vi "Display Soft Trigger Status.vi"(11 "Soft Trig enum":T1(ring)) -> (3 "String":string)   [LabVIEW 2016, in "CML UI.lvlib"]
uses:
  CML UI.lvlib
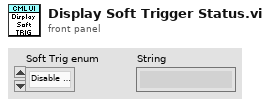
[diagram p1: front panel]
types:
  T1 = enum16{"Disable Soft Trigger", "Enable Soft Trigger"}
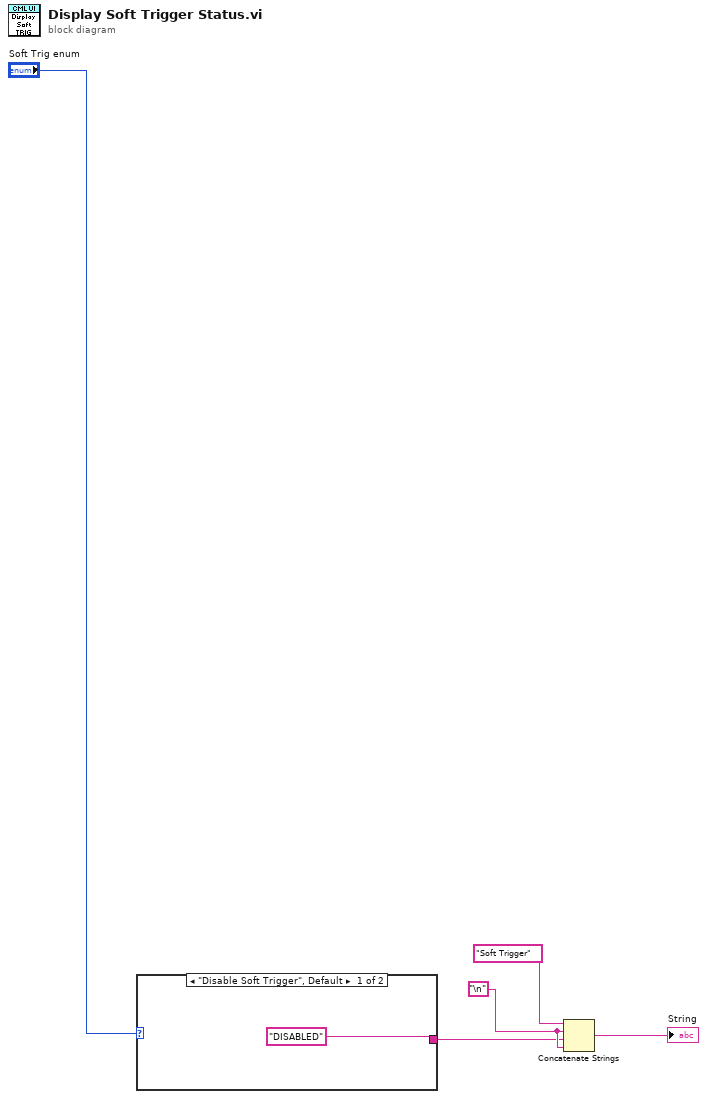
[diagram p0: block diagram]
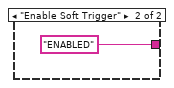
[diagram p2: hidden frame]
diagram:
  w3 = "\n"
  n1 = case shown="\"Disable Soft Trigger\", Default" "Soft Trig enum" {
    tunnel: ["DISABLED" "ENABLED"] -> w2
    frame "Disable Soft Trigger", Default {
    }
    frame "Enable Soft Trigger" {
    }
  }
  n2 = Concatenate Strings("Soft Trigger" ("string"), w3, w2, w3) -> (→"String":string)
